vi "FTW-Request-Ask.vi"(0 "FTW-Request In":refnum<class "FTW-Request.lvclass">, 5 "Header":string, 7 "Body":string, 9 "Timeout":i32=1000 format="%dmsec", 11 "error in":errorcluster) -> (4 "FTW-Request Out":refnum<class "FTW-Request.lvclass">, 6 "Response Header":string, 8 "Response Body":string, 10 "Timed out?":bool, 13 "Response Metadata":string, 14 "Roundtrip Time":dbl format="%.6fsec", 15 "error out":errorcluster)   [LabVIEW 2013, in "FTW-Request.lvclass"]
uses:
  FTW-Request.lvclass
  FTW-Request.lvclass/FTW-Request.ctl
  Endpoint/FTW-Endpoint.lvclass
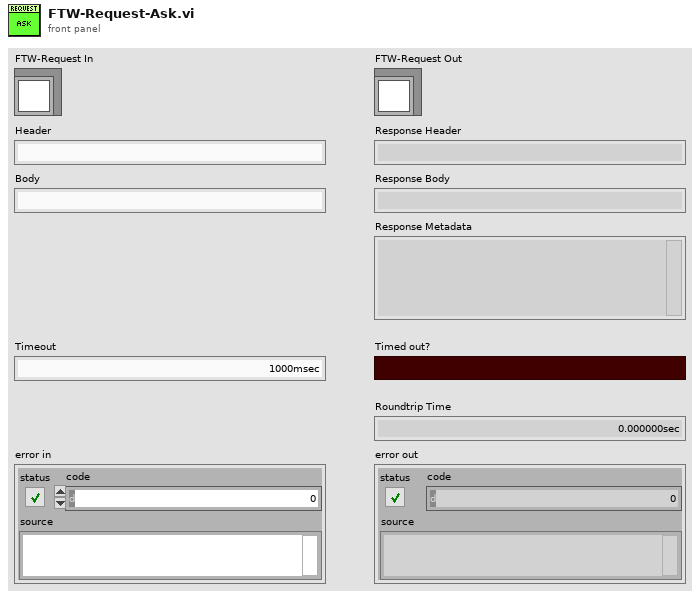
[diagram p1: front panel]
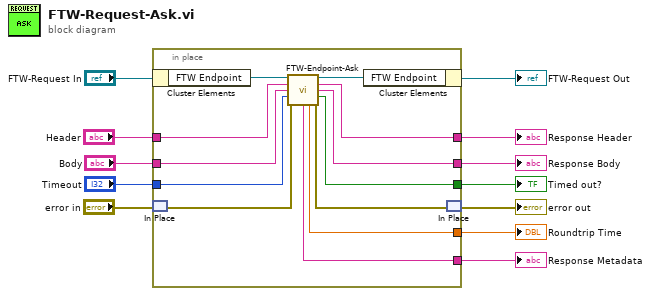
[diagram p0: block diagram]
diagram:
  n1 = in-place {
    in-place-border: "Header" -> [w20]
    in-place-border: "Body" -> [w19]
    in-place-border: "Timeout" -> [w18]
    in-place-border: [w16] -> w2
    in-place-border: [w17] -> w3
    in-place-border: [w15] -> w5
    in-place-border: [w14] -> w4
    in-place-border: [w13] -> w1
    n2 = in-place-cluster #1("FTW-Request In") -> ("FTW Endpoint"=w22:refnum<class "FTW-Endpoint.lvclass">)
    n3 = in-place-match #2("error in") -> (w24:errorcluster)
    n4 = call-dynamic "FTW-Endpoint-Ask.vi"("FTW Endpoint"=w22, "Request Header"=w20, "Request Body"=w19, "Timeout"=w18, "error in"=w24) -> ("FTW Endpoint out"=w21:refnum<class "FTW-Endpoint.lvclass">, "Response Header"=w17:string, "Response Body"=w16:string, "Timed out?"=w15:bool, "Response Metadata"=w13:string, "Roundtrip Time"=w14:dbl, "error out"=w23:errorcluster)  [unwired: 4 in]
    n5 = in-place-cluster #1("FTW Endpoint"=w21) -> (→"FTW-Request Out":refnum<class "FTW-Request.lvclass">)
    n6 = in-place-match #2(w23) -> (→"error out":errorcluster)
  }
  "Response Header" <- w3
  "Response Body" <- w2
  "Timed out?" <- w5
  "Roundtrip Time" <- w4
  "Response Metadata" <- w1
